vi "Get Sensor Block.vi"(11 "Select Probe":i32) -> (2 "Sensor Block":T1 {"SensorCfgParams Array"."CalibrCoefArray" format="%#.12g"})   [LabVIEW 2015, in "Tool Cfg.lvlib"]
uses:
  Tool Cfg.lvlib
  _Sensor Block Cluster--typedef.ctl
  _SensorConfigParams Cluster--typedef.ctl
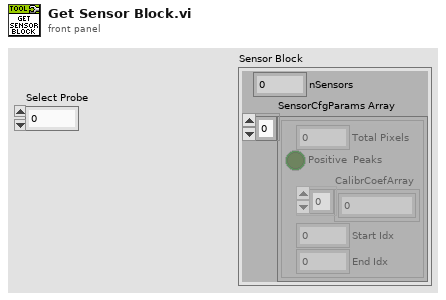
[diagram p1: front panel]
types:
  T1 = typedef "Tool Cfg.lvlib/_Sensor Block Cluster--typedef.ctl" = cluster{"nSensors":u16, "SensorCfgParams Array":T2[]}
  T2 = typedef "Tool Cfg.lvlib/_SensorConfigParams Cluster--typedef.ctl" = cluster{"Total Pixels":u16, "Positive  Peaks":bool, "CalibrCoefArray":dbl[], "Start Idx":u16, "End Idx":u16}
  T3 = typedef "Tool Cfg.lvlib/_ProbeConfigParams Cluster--typedef.ctl" = cluster{"Name":string, "Laser Init Pwr":u16, "Laser Gain":u8, "Integ Count":u16, "Meas. Range":sgl, "Angle":sgl, "Probe Offset":sgl, "Sensor Block":T1}
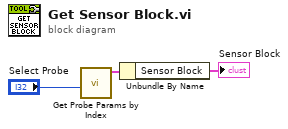
[diagram p0: block diagram]
diagram:
  n1 = call "Get Probe Params by Index.vi"("Probe Select"="Select Probe") -> ("Probe Cfg Params"=w3:T3)  [unwired: 10 in]
  n2 = Unbundle By Name(w3) -> ("Sensor Block"=→"Sensor Block":T1)
